vi "ErrorManager.vi"(5 "This error short circuits?":bool, 7 "This error occurred?":bool, 8 "ErrorInfo In":T1, 11 "XError Cluster":T3) -> (0 "ErrorInfo Out":T1)   [LabVIEW 2020, in "NI_XNodeSupport.lvlib"]
doc: "Manages error information for you in ListErrors so that you can efficiently compute your errors. See the design pattern posted on the XNode developers forum for how to use."
uses:
  NI_XNodeSupport.lvlib
  XNodeError3.ctl
  XNodeString.ctl
  ErrorInfo.ctl
  XNodeError3Array.ctl
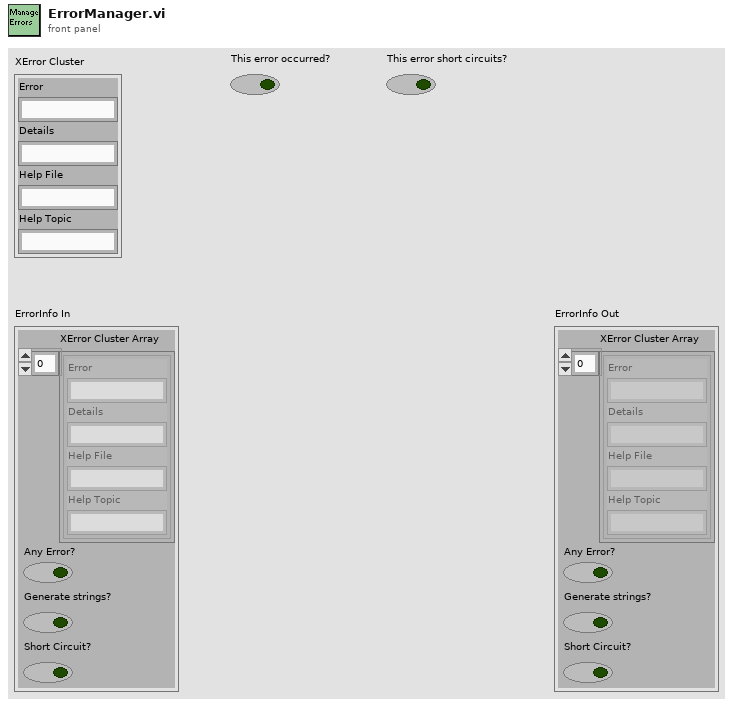
[diagram p1: front panel]
types:
  T1 = typedef "NI_XNodeSupport.lvlib/ErrorInfo.ctl" = cluster{"XError Cluster Array":T2, "Any Error?":bool, "Generate strings?":bool, "Short Circuit?":bool}
  T2 = typedef "NI_XNodeSupport.lvlib/XNodeError3Array.ctl" = T3[]
  T3 = typedef "NI_XNodeSupport.lvlib/XNodeError3.ctl" = cluster{"Error":T4, "Details":T4, "Help File":T4, "Help Topic":T4}
  T4 = typedef "NI_XNodeSupport.lvlib/XNodeString.ctl" = string
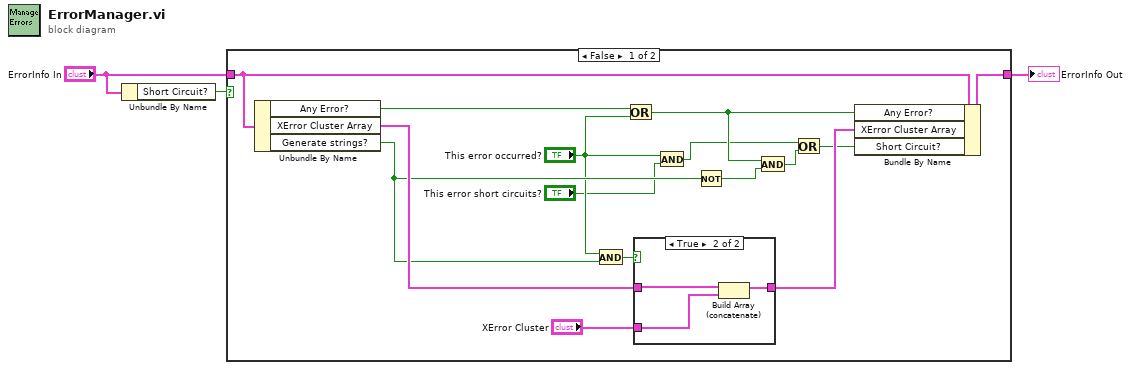
[diagram p0: block diagram]
diagram:
  n1 = Unbundle By Name("ErrorInfo In") -> ("Short Circuit?"=w1:bool)
  n2 = case shown="False" w1 {
    tunnel: "ErrorInfo In" -> [w14 w23]
    tunnel: [w12 w23] -> w3
    frame False {
      n3 = Unbundle By Name(w14) -> ("Any Error?"=w16:bool, "XError Cluster Array"=w15:T2, "Generate strings?"=w11:bool)
      n4 = And(x="This error occurred?", y=w11) -> (x .and. y?=w18:bool)
      n5 = Or(x=w16, y="This error occurred?") -> (x .or. y?=w10:bool)
      n6 = case shown="True" w18 {
        tunnel: w15 -> [w19 w22]
        tunnel: "XError Cluster" -> [_ w21]
        tunnel: [w19 w20] -> w13
        frame False {
        }
        frame True {
          n7 = Build Array (concatenate)(w22, w21) -> (w20:T2)
        }
      }
      n8 = And(x="This error occurred?", y="This error short circuits?") -> (x .and. y?=w5:bool)
      n9 = Not(x=w11) -> (.not. x?=w9:bool)
      n10 = And(x=w10, y=w9) -> (x .and. y?=w6:bool)
      n11 = Or(x=w5, y=w6) -> (x .or. y?=w4:bool)
      n12 = Bundle By Name(cluster=w14, "Any Error?"=w10, "XError Cluster Array"=w13, "Short Circuit?"=w4) -> (w12:T1)
    }
    frame True {
    }
  }
  "ErrorInfo Out" <- w3
